vi "Mode Localization.vi"(8 "Function":T1) -> (0 "Localized Mode":i32(ring) items=["Sine"=0, "Square"=1, "Ramp"=2, "Noise"=3, "DC"=4, "Triangle"=5, "Pulse"=6, "Sinc"=11, "D-Lorentz"=12, "Gaussian"=13, "Expo Fall"=14, "Expo Rise"=15, "Haversine"=16])   [LabVIEW 2019]
uses:
  builds/Instruments/FunctionGenerator.lvlibp/Custom Controls/WaveformMode.ctl
  builds/Instruments/FunctionGenerator.lvlibp/Library/FunctionGenerator.lvclass
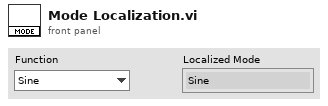
[diagram p1: front panel]
types:
  T1 = typedef "FunctionGenerator.lvlibp/FunctionGenerator.lvclass/WaveformMode.ctl" = enum16{"Sine", "Square", "Ramp", "Pulse", "Arbitrary", "Triangle", "Noise", "DC"}
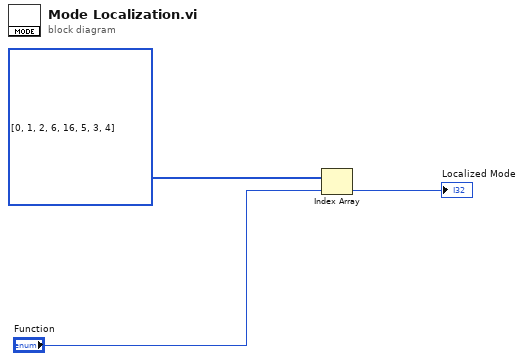
[diagram p0: block diagram]
diagram:
  w3 = i32[] [0, 1, 2, 6, 16, 5, 3, 4] items=["Sine"=0, "Square"=1, "Ramp"=2, "Noise"=3, "DC"=4, "Triangle"=5, "Pulse"=6, "Sinc"=11, "D-Lorentz"=12, "Gaussian"=13, "Expo Fall"=14, "Expo Rise"=15, "Haversine"=16]
  n1 = Index Array(array=w3, index="Function") -> (element=→"Localized Mode":i32)
